vi "Serialize Class.vi"(7 "formatter":refnum<class "Formatter.lvclass">, 8 "error in":errorcluster, 9 "Port":refnum<visa-resource-name>, 10 "Name":string, 11 "Serial IO in":refnum<class "Serial IO.lvclass">) -> (0 "error out":errorcluster, 2 "JSON String":string, 3 "Serial IO out":refnum<class "Serial IO.lvclass">)   [LabVIEW 2012]
uses:
  <userlib>/Serialization/Serializer/Serializer.lvclass
  <userlib>/Serialization/JSON Serializer/JSON Serializer.lvclass
  Serial IO.lvclass
  <userlib>/Serialization/Formatter/Formatter.lvclass
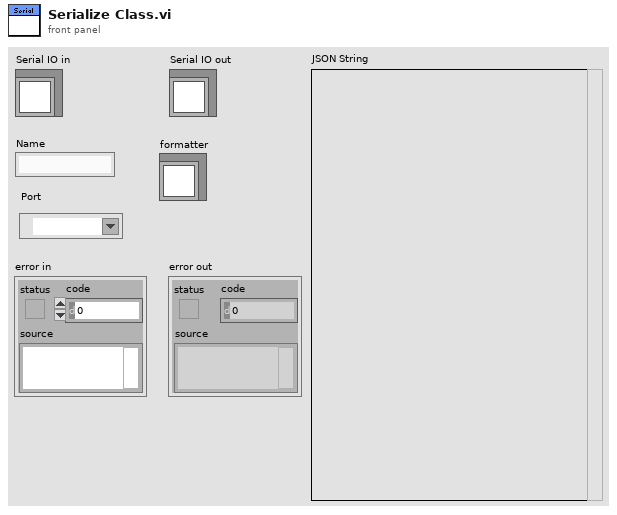
[diagram p1: front panel]
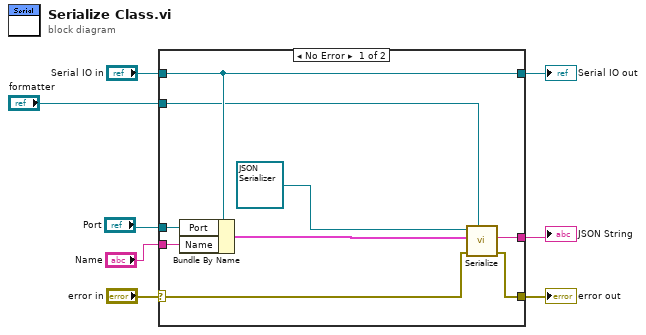
[diagram p0: block diagram]
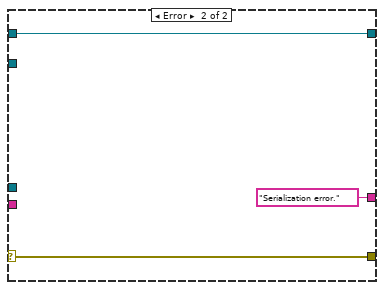
[diagram p2: hidden frame]
diagram:
  n1 = case shown="No Error" "error in" {
    selector: "error in" -> [w12 w20]
    tunnel: [w10 w20] -> w7
    tunnel: [w14 w19] -> w5
    tunnel: "Serial IO in" -> [w14 w19]
    tunnel: "Port" -> [w17 _]
    tunnel: "Name" -> [w16 _]
    tunnel: [w11 "Serialization error." ("String")] -> w2
    tunnel: "formatter" -> [w9 _]
    frame No Error {
      n2 = Bundle By Name(cluster=w14, "Port"=w17, "Name"=w16) -> (w15:cluster{})
      n3 = call <userlib>:"Serialize.vi"("Formatter (defaults)"=w9, "error in (no error)"=w12, "Serializable"=w15, "Serializer"=refnum<class "JSON Serializer.lvclass"> refnum ("JSON Serializer.lvclass")) -> ("error out"=w10:errorcluster, "String"=w11:string)  [unwired: 5 in, 1 out]
    }
    frame Error {
    }
  }
  "error out" <- w7
  "Serial IO out" <- w5
  "JSON String" <- w2
